vi "BL_GetHardConf.vi"(8 "error in (no error)":errorcluster, 10 "Channel":u8, 11 "Potentiostat Galvanostat in":refnum<class "Potentiostat Galvanostat.lvclass">) -> (0 "error out":errorcluster, 1 "Hardware Configuration":T1 {"Instrument ground" items=["Grounded Mode", "Floating Mode"]; "Electrode connection" items=["Standard connection", "CE to ground connection", "WE to ground connection", "High Voltage Connection"]}, 2 "Channel":u8, 3 "Potentiostat Galvanostat out":refnum<class "Potentiostat Galvanostat.lvclass">)   [LabVIEW 2018, in "Potentiostat Galvanostat.lvclass"]
doc: "This function return in pHardConf the hardware configuration of the\nchannel ch. The hardware configuration is the electrode connection\nand the instrument ground.\nThis function must be used only with SP-300 series."
uses:
  Potentiostat Galvanostat.lvclass
  Controls/Hardware Configuration.ctl
  Controls/Electrode Connection.ctl
  Controls/Electrode Mode.ctl
  Potentiostat Galvanostat.lvclass/Potentiostat Galvanostat.ctl
  BL_GetErrorMsg.vi
  <vilib>/Utility/error.llb/Error Cluster From Error Code.vi
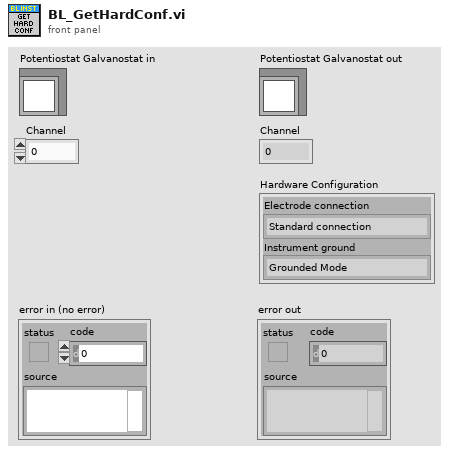
[diagram p1: front panel]
types:
  T1 = typedef "Potentiostat Galvanostat.lvclass/Hardware Configuration.ctl" = cluster{"Electrode connection":T2, "Instrument ground":T3}
  T2 = typedef "Potentiostat Galvanostat.lvclass/Electrode Connection.ctl" = i32
  T3 = typedef "Potentiostat Galvanostat.lvclass/Electrode Mode.ctl" = i32
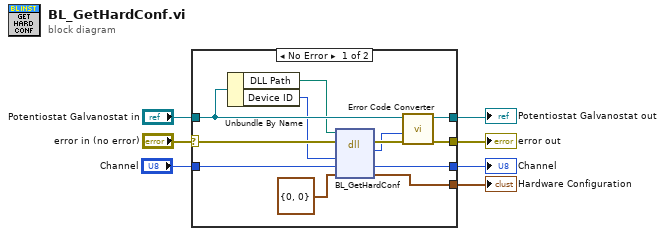
[diagram p0: block diagram]
diagram:
  n1 = case shown="No Error" "error in (no error)" {
    selector: "error in (no error)" -> [w15 w21]
    tunnel: [w19 w21] -> w6
    tunnel: [w18 w20] -> w4
    tunnel: "Potentiostat Galvanostat in" -> [w17 w20]
    tunnel: "Channel" -> [w14 _]
    tunnel: [w11 _] -> w1
    tunnel: [w10 _] -> w2
    frame No Error {
      n2 = Unbundle By Name(w17) -> ("DLL Path"=w12:path, "Device ID"=w13:i32)
      n3 = dll-call lib="C:/Program Files (x86)/National Instruments/LabVIEW 2018/user.lib/EClib/EClib.*" fn="BL_GetHardConf"(path in=w12, error in=w15, "Device ID"=w13, "Channel"=w14, "Hardware Configuration"=T1 {"Electrode connection"=0, "Instrument ground"=0}) -> (error out=w9:errorcluster, "Error Code"=w8:i32, "Channel"=w10:u8, "Hardware Configuration"=w11:T1)  [unwired: 2 in, 1 out]
      n4 = call "Error Code Converter.vi"("error in (no error)"=w9, "Error Code"=w8, "Potentiostat Galvanostat in"=w17) -> ("error out"=w19:errorcluster, "Potentiostat Galvanostat out"=w18:refnum<class "Potentiostat Galvanostat.lvclass">)  [unwired: 7 in]
    }
    frame Error {
    }
  }
  "error out" <- w6
  "Potentiostat Galvanostat out" <- w4
  "Channel" <- w2
  "Hardware Configuration" <- w1
